vi "Loop_SM.vi"() -> ()   [LabVIEW 2017, in "Arm.lvlib"]
uses:
  Arm.lvlib
  CLUSTER_CMD_SM_Lift_Rotate.ctl
  ENUM_SM_Rotate_Positions.ctl
  _SHARE ALL/TypeDef Share All/CLUSTER_TalonInput.ctl
  System Drivers/Phoenix-LabVIEW/Motor Controller/Controls/CTRE_Phoenix_MotorControl_ControlMode.ctl
  TypeDef/CLUSTER_PID.ctl
  ENUM_SM_State.ctl
  CLUSTER_ACT_Lift Output.ctl
  _SHARE ALL/RoboRio Share All/SRX Share All/TypeDefs SRX/Cluster_SRX_General Data.ctl
  _SHARE ALL/RoboRio Share All/SRX Share All/TypeDefs SRX/Cluster_SRX_Common Runtime Data.ctl
  _SHARE ALL/RoboRio Share All/SRX Share All/TypeDefs SRX/Cluster_SRX_Error Calculations.ctl
  _SHARE ALL/RoboRio Share All/SRX Share All/TypeDefs SRX/Cluster_SRX_Voltage Out Data.ctl
  _SHARE ALL/RoboRio Share All/SRX Share All/TypeDefs SRX/Cluster_SRX_Sensor Out Data.ctl
  _SHARE ALL/RoboRio Share All/SRX Share All/TypeDefs SRX/Cluster_SRX_Sensor Quad Data.ctl
  _SHARE ALL/RoboRio Share All/SRX Share All/TypeDefs SRX/Cluster_SRX_Analog In Data.ctl
  _SHARE ALL/RoboRio Share All/SRX Share All/TypeDefs SRX/Cluster_SRX_PWM Sensor Data.ctl
  _SHARE ALL/RoboRio Share All/SRX Share All/TypeDefs SRX/Cluster_SRX_F and R Limit Indicators.ctl
  ENUM_SM_Action.ctl
  Globals/Global_Device_IDs.vi
  _SHARE ALL/Global Share All/Global_STOP.vi
  Global_CMD.vi
  Global_ACT Write_Data Out.vi
  Global_SM Write_Data Out.vi
panel:
  out "State":T1
  out "SM Output":T2 {"Talon Mode" items=["PercentOutput"=0, "Position"=1, "Velocity"=2, "Current"=3, "Follower"=5, "MotionProfile"=6, "MotionMagic"=7, "MotionMagicArc"=8, "MotionProfileArc"=10, "Disabled"=15]}
  out "SM CMD Input":T5={"Enable System"=TRUE, "Rotate Position"=enum."Neutral: 3340", "Manual Velocity"=0.0, "Manual Mode"=FALSE, "Manual Override"=FALSE}
  out "Cycle Time (S)":dbl format="%.3g"
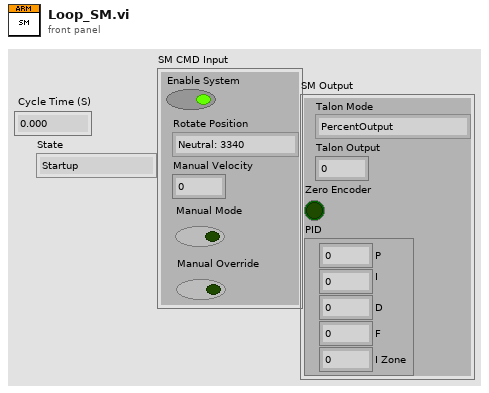
[diagram p1: front panel]
types:
  T1 = typedef "Arm.lvlib/ENUM_SM_State.ctl" = enum16{"Startup", "Idle", "F_Manual", "Manual", "Position - Moving", "Position - Holding", "Shutdown"}
  T2 = typedef "CLUSTER_TalonInput.ctl" = cluster{"Talon Mode":T3, "Talon Output":dbl, "Zero Encoder":bool, "PID":T4}
  T3 = typedef "CTRE_Phoenix_MotorControl_ControlMode.ctl" = u16
  T4 = typedef "CLUSTER_PID.ctl" = cluster{"P":dbl, "I":dbl, "D":dbl, "F":dbl, "I Zone":dbl}
  T5 = typedef "Arm.lvlib/CLUSTER_CMD_SM_Lift_Rotate.ctl" = cluster{"Enable System":bool, "Rotate Position":T6, "Manual Velocity":dbl, "Manual Mode":bool, "Manual Override":bool}
  T6 = typedef "Arm.lvlib/ENUM_SM_Rotate_Positions.ctl" = enum16{"Neutral: 3340", "Pickup: 0", "Switch: 0", "Scale: 0", "Climb: 0"}
  T7 = typedef "Arm.lvlib/CLUSTER_ACT_Lift Output.ctl" = cluster{"Device Info Out":T8, "Common Runtime Data Out":T9, "Quad Sensor Data Out":T13, "Analog Sensor Data Out":T14, "PWM Data Out":T15, "Hard Limits Out":T16}
  T8 = typedef "Cluster_SRX_General Data.ctl" = cluster{"Device ID":i32, "Firmware Version":i32, "Inverted?":bool, "Has Reset Occurred?":bool}
  T9 = typedef "Cluster_SRX_Common Runtime Data.ctl" = cluster{"Calc":T10, "Voltage ":T11, "Sensor":T12, "Current":dbl, "Temp":dbl}
  T10 = typedef "Cluster_SRX_Error Calculations.ctl" = cluster{"Error":i32, "D-Error":dbl, "I-Acc":dbl}
  T11 = typedef "Cluster_SRX_Voltage Out Data.ctl" = cluster{"Percent":dbl, "Output":dbl, "Bus":dbl}
  T12 = typedef "Cluster_SRX_Sensor Out Data.ctl" = cluster{"Pos":i32, "Vel":i32}
  T13 = typedef "Cluster_SRX_Sensor Quad Data.ctl" = cluster{"Position":i32, "Velocity":i32, "Quad A Pin":bool, "Quad B Pin":bool, "Quad Idx Pin":bool}
  T14 = typedef "Cluster_SRX_Analog In Data.ctl" = cluster{"WithOv":i32, "Raw":i32, "Velocity":i32}
  T15 = typedef "Cluster_SRX_PWM Sensor Data.ctl" = cluster{"Position":i32, "Velocity":i32, "High(us)":i32, "Period(us)":i32}
  T16 = typedef "Cluster_SRX_F and R Limit Indicators.ctl" = cluster{"Forward Closed?":bool, "Reverse Closed?":bool}
  T17 = typedef "Arm.lvlib/ENUM_SM_Action.ctl" = enum16{"No Action", "Reset Time", "Reset All", "Reset Encoder", "F_Manual", "Manual", "Position", "Set PID 1", "Disable Motor"}
  T18 = typedef "CLUSTER_Arm_Device_IDs.ctl" = cluster{"Master":T19, "Slave":T19, "Up PIDF":T27, "Down PIDF":T27}
  T19 = typedef "CLUSTER_Talon_Setup.ctl" = cluster{"Open Data":T20, "Current Config Data":T21, "Sensor Config":T22, "Hard Limits":T24, "Motion Magic Config Data":T26, "PIDF":T27, "Maximum Integral Accumulator Value":dbl, "AllowableClosedLoop":i32, "Limits":T28, "Output Config":T29}
  T20 = typedef "Cluster_SRX_OPEN Data.ctl" = cluster{"SRX ID":u8, "Invert Output":bool}
  T21 = typedef "Cluster_SRX_Current Config.ctl" = cluster{"Enable Current Limit?":bool, "Peak Current (Amps)":i32, "Peak Current Maximum Duration (ms)":i32, "Continuous Current Limit (Amps)":i32}
  T22 = typedef "Cluster_SRX_Sensor Config.ctl" = cluster{"Feedback Device":T23, "PhaseSensor":bool}
  T23 = typedef "CTRE_Phoenix_MotorControl_FeedbackDevice.ctl" = i8
  T24 = typedef "Cluster_SRX_Config Hard Limits.ctl" = cluster{"Fwd Enable":bool, "Rev Enable":bool, "Fwd NO-NC":T25, "Rev NO-NC":T25}
  T25 = typedef "CTRE_Phoenix_MotorControl_LimitSwitchNormal.ctl" = enum16{"Normally Open", "Normally Closed", "Disabled"}
  T26 = typedef "Cluster_SRX_Motion Magic Config Data.ctl" = cluster{"Cruise Velocity":i32, "Acceleration":i32}
  T27 = typedef "Cluster_SRX_PIDF.ctl" = cluster{"P":dbl, "I":dbl, "D":dbl, "F":dbl, "I Zone":dbl}
  T28 = typedef "Cluster_SRX_Config Soft Limits.ctl" = cluster{"Max":i32, "Min":i32, "Max Enable":bool, "Min Enable":bool}
  T29 = typedef "Cluster_SRX_Config Voltage Output.ctl" = cluster{"Invert?":bool, "Neutral Mode":T30, "Deadband (-1to1)":dbl, "Ramp Time Off to Full (S)":dbl, "Peak  (-1to1)":T31, "Nominal  (-1to1)":T31}
  T30 = typedef "CTRE_Phoenix_MotorControl_NeutralMode.ctl" = enum8{"EEPROMSetting", "Override to Coast", "Override to Brake"}
  T31 = typedef "Cluster_SRX_Forward and Reverse.ctl" = cluster{"Forward":dbl, "Reverse":dbl}
  T32 = cluster{"State":T1, "Previous State":T1, "Current Time":timestamp, "Previous Time":timestamp, "Start Time":timestamp, "Target Time (ms)":u32, "Cycle Time(S)":dbl, "Arm_Output":T7, "SM CMD Input":T5, "SM Output":T2, "Arm Setup":T18, "Manual Counter":i32}
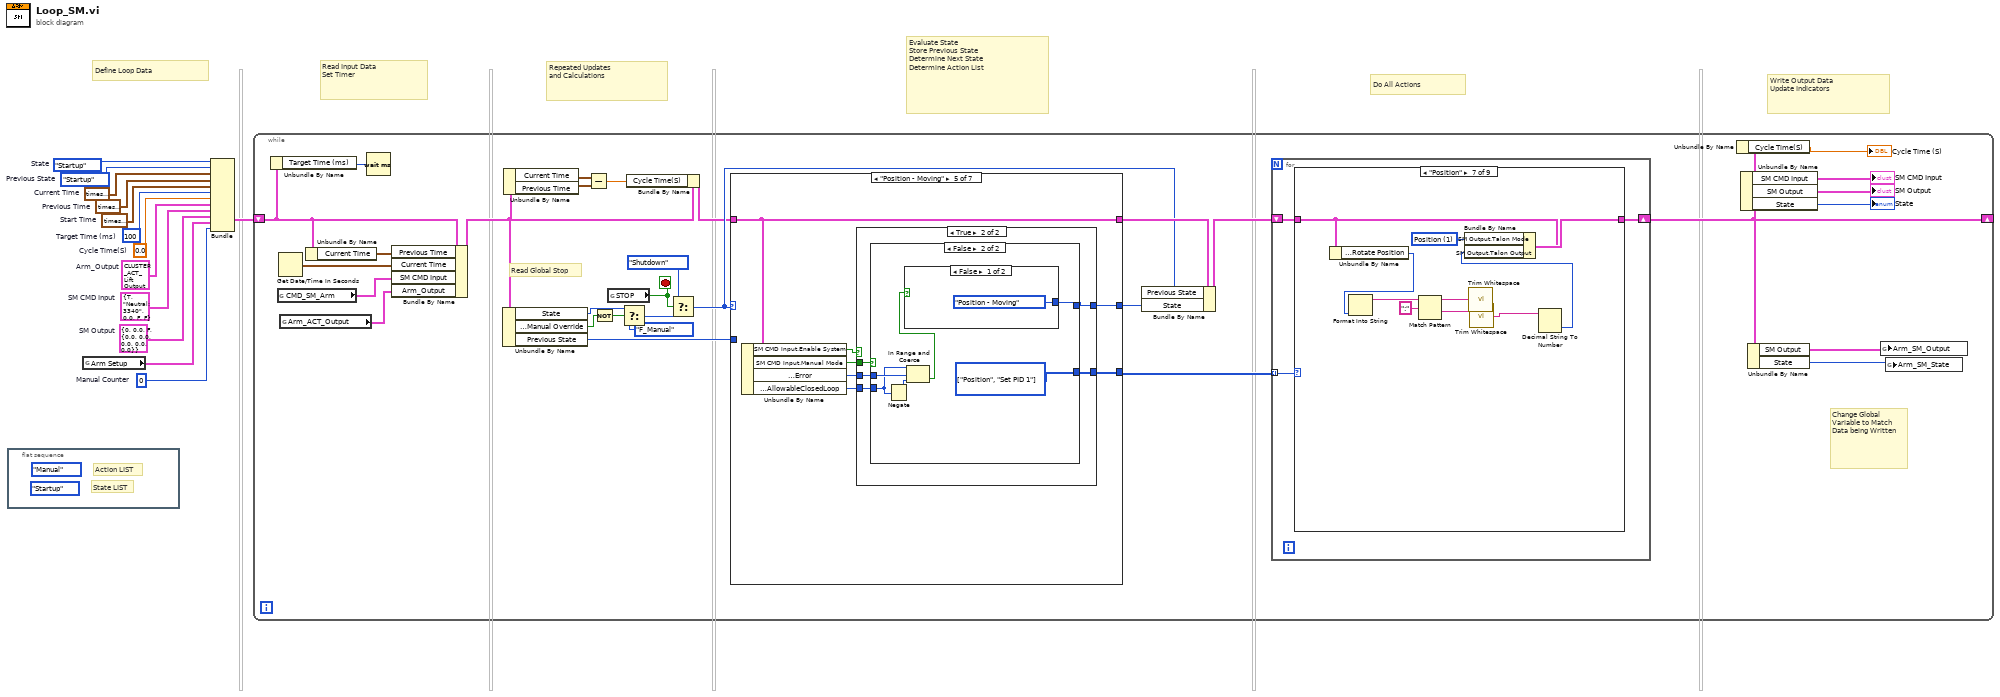
[diagram p0: block diagram]
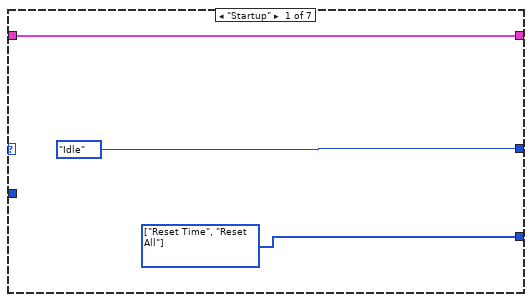
[diagram p2: hidden frame]
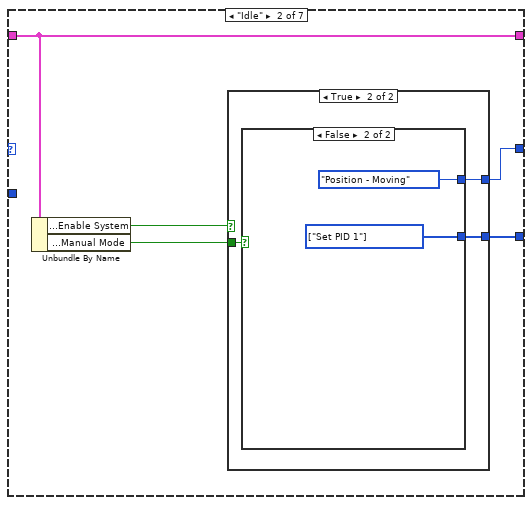
[diagram p3: hidden frame]
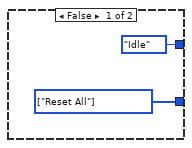
[diagram p4: hidden frame]
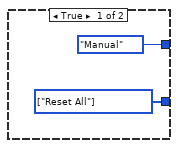
[diagram p5: hidden frame]
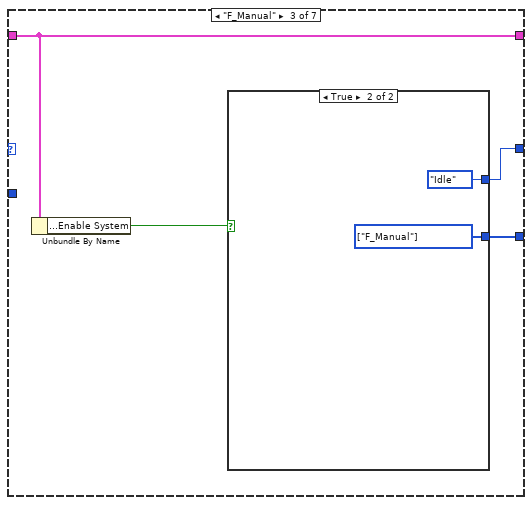
[diagram p6: hidden frame]
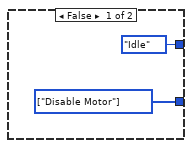
[diagram p7: hidden frame]
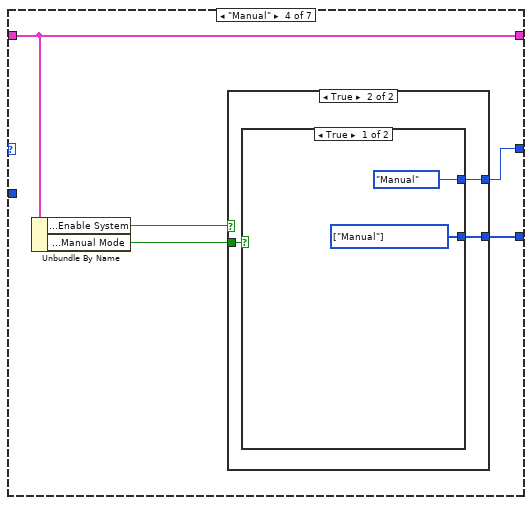
[diagram p8: hidden frame]
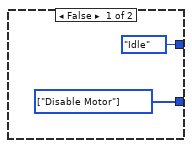
[diagram p9: hidden frame]
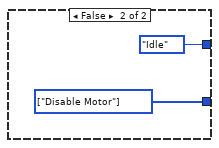
[diagram p10: hidden frame]
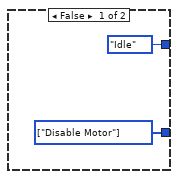
[diagram p11: hidden frame]
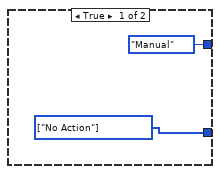
[diagram p12: hidden frame]
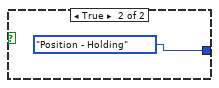
[diagram p13: hidden frame]
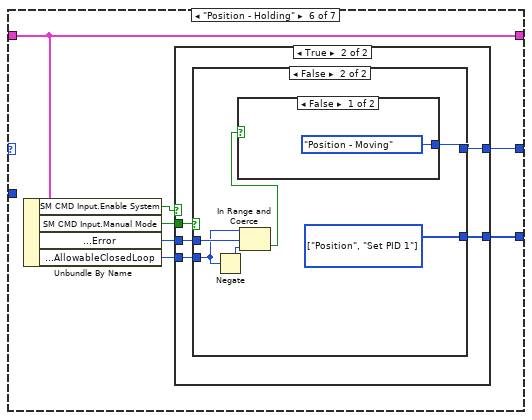
[diagram p14: hidden frame]
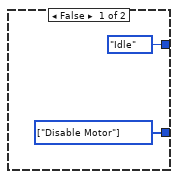
[diagram p15: hidden frame]
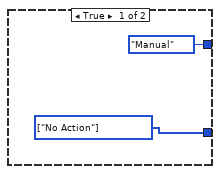
[diagram p16: hidden frame]
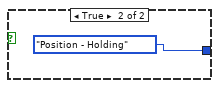
[diagram p17: hidden frame]
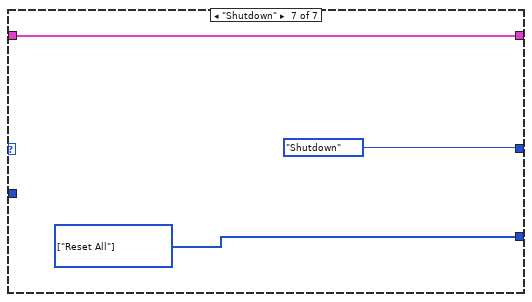
[diagram p18: hidden frame]
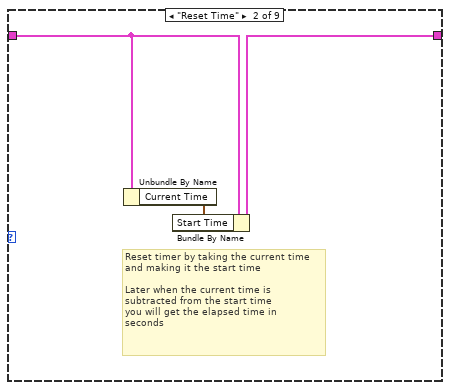
[diagram p20: hidden frame]
diagram:
  w1 = 0  # Manual Counter
  w3 = T2 {"Talon Mode"=0, "Talon Output"=0.0, "Zero Encoder"=FALSE, "PID"={"P"=0.0, "I"=0.0, "D"=0.0, "F"=0.0, "I Zone"=0.0}}  # SM Output
  w4 = T5 {"Enable System"=TRUE, "Rotate Position"=enum."Neutral: 3340", "Manual Velocity"=0.0, "Manual Mode"=FALSE, "Manual Override"=FALSE}  # SM CMD Input
  w5 = T7 {"Device Info Out"={"Device ID"=0, "Firmware Version"=0, "Inverted?"=FALSE, "Has Reset Occurred?"=FALSE}, "Common Runtime Data Out"={"Calc"={"Error"=0, "D-Error"=0.0, "I-Acc"=0.0}, "Voltage "={"Percent"=0.0, "Output"=0.0, "Bus"=0.0}, "Sensor"={"Pos"=0, "Vel"=0}, "Current"=0.0, "Temp"=0.0}, "Quad Sensor Data Out"={"Position"=0, "Velocity"=0, "Quad A Pin"=FALSE, "Quad B Pin"=FALSE, "Quad Idx Pin"=FALSE}, "Analog Sensor Data Out"={"WithOv"=0, "Raw"=0, "Velocity"=0}, "PWM Data Out"={"Position"=0, "Velocity"=0, "High(us)"=0, "Period(us)"=0}, "Hard Limits Out"={"Forward Closed?"=FALSE, "Reverse Closed?"=FALSE}}  # Arm_Output
  w6 = 0.0  # Cycle Time(S)
  w7 = ENUM_SM_State."Startup"  # Previous State
  w8 = timestamp(0 s since 1904-01-01)  # Previous Time
  w9 = u32 100  # Target Time (ms)
  w10 = timestamp(0 s since 1904-01-01)  # Start Time
  w11 = timestamp(0 s since 1904-01-01)  # Current Time
  w12 = ENUM_SM_State."Startup"  # State
  # "Define Loop Data"
  # "Repeated Updates\nand Calculations"
  # "Read Input Data\nSet Timer"
  # "Evaluate State\nStore Previous State\nDetermine Next State\nDetermine Action List"
  # "Do All Actions"
  # "Write Output Data\nUpdate Indicators"
  n1 = flat-sequence {
    frame #0 {
      (unwired) ENUM_SM_State."Startup" ("State")
      (unwired) ENUM_SM_Action."Manual" ("Action")
      # "State LIST"
      # "Action LIST"
    }
  }
  n2 = global read "Global_Device_IDs.vi" "Arm Setup"() -> (w2:T18)
  n3 = Bundle("State"=w12, "Previous State"=w7, "Current Time"=w11, "Previous Time"=w8, "Start Time"=w10, "Target Time (ms)"=w9, "Cycle Time(S)"=w6, "Arm_Output"=w5, "SM CMD Input"=w4, "SM Output"=w3, "Arm Setup"=w2, "Manual Counter"=w1) -> (w13:T32)  [unwired: 1 in]
  n4 = while {
    shift-right: [w35] -> _
    shift-left: w13 -> [w37]
    stop <- w41 stop-if-true
    # "Change Global\nVariable to Match\nData being Written"
    # "Read Global Stop"
    n5 = Unbundle By Name(w37) -> ("Target Time (ms)"=w39:u32)
    n6 = global read "Global_CMD.vi" "CMD_SM_Arm"() -> (w27:T5)
    n7 = Get Date/Time In Seconds() -> (seconds since 1Jan1904=w44:timestamp)
    n8 = global read "Global_ACT Write_Data Out.vi" "Arm_ACT_Output"() -> (w26:T7)
    n9 = Unbundle By Name(w37) -> ("Current Time"=w38:timestamp)
    n10 = Wait (ms)(milliseconds to wait=w39) -> ()  [unwired: 1 out]
    n11 = Bundle By Name(cluster=w37, "Previous Time"=w38, "Current Time"=w44, "SM CMD Input"=w27, "Arm_Output"=w26) -> (w31:T32)
    n12 = Unbundle By Name(w31) -> ("State"=w17:T1, "SM CMD Input.Manual Override"=w18:bool, "Previous State"=w19:T1)
    n13 = Unbundle By Name(w31) -> ("Current Time"=w32:timestamp, "Previous Time"=w33:timestamp)
    n14 = Subtract(x=w32, y=w33) -> (x-y=w29:dbl)
    n15 = Not(x=w18) -> (.not. x?=w14:bool)
    n16 = global read "Global_STOP.vi" "STOP"() -> (w41:bool)
    n17 = Select(t=w17, s=w14, f=ENUM_SM_State."F_Manual") -> (s? t:f=w15:T1)
    n18 = Bundle By Name(cluster=w31, "Cycle Time(S)"=w29) -> (w30:T32)
    n19 = Select(t=ENUM_SM_State."Shutdown" ("State"), s=w41, f=w15) -> (s? t:f=w36:T1)
    n20 = case shown="\"Position - Moving\"" w36 {
      tunnel: w30 -> [w47 w52 w65 w74 w90 w114 w134]
      tunnel: [w47 w52 w65 w74 w90 w114 w134] -> w42
      tunnel: [w46 w48 w62 w70 w86 w110 w133] -> w28
      tunnel: [ENUM_SM_State."Idle" ("State") w49 w63 w71 w85 w109 ENUM_SM_State."Shutdown" ("State")] -> w25
      tunnel: w19 -> [_ _ _ _ _ _ _]
      frame "Startup" {
        w46 = T17[] [enum."Reset Time", enum."Reset All"] items=["No Action", "Reset Time", "Reset All", "Reset Encoder", "F_Manual", "Manual", "Position", "Set PID 1", "Disable Motor"] ("Actions")
      }
      frame "Idle" {
        n21 = Unbundle By Name(w52) -> ("SM CMD Input.Enable System"=w51:bool, "SM CMD Input.Manual Mode"=w50:bool)
        n22 = case shown="True" w51 {
          tunnel: w50 -> [_ w57]
          tunnel: [ENUM_SM_State."Idle" ("State") w56] -> w49
          tunnel: [w53 w55] -> w48
          frame False {
            w53 = T17[] [enum."Reset All"] items=["No Action", "Reset Time", "Reset All", "Reset Encoder", "F_Manual", "Manual", "Position", "Set PID 1", "Disable Motor"] ("Actions")
          }
          frame True {
            n23 = case shown="False" w57 {
              tunnel: [ENUM_SM_State."Manual" ("State") ENUM_SM_State."Position - Moving" ("State")] -> w56
              tunnel: [w58 w60] -> w55
              frame True {
                w58 = T17[] [enum."Reset All"] items=["No Action", "Reset Time", "Reset All", "Reset Encoder", "F_Manual", "Manual", "Position", "Set PID 1", "Disable Motor"] ("Actions")
              }
              frame False {
                w60 = T17[] [enum."Set PID 1"] items=["No Action", "Reset Time", "Reset All", "Reset Encoder", "F_Manual", "Manual", "Position", "Set PID 1", "Disable Motor"] ("Actions")
              }
            }
          }
        }
      }
      frame "F_Manual" {
        n24 = Unbundle By Name(w65) -> ("SM CMD Input.Enable System"=w64:bool)
        n25 = case shown="True" w64 {
          tunnel: [ENUM_SM_State."Idle" ("State") ENUM_SM_State."Idle" ("State")] -> w63
          tunnel: [w66 w68] -> w62
          frame False {
            w66 = T17[] [enum."Disable Motor"] items=["No Action", "Reset Time", "Reset All", "Reset Encoder", "F_Manual", "Manual", "Position", "Set PID 1", "Disable Motor"] ("Actions")
          }
          frame True {
            w68 = T17[] [enum."F_Manual"] items=["No Action", "Reset Time", "Reset All", "Reset Encoder", "F_Manual", "Manual", "Position", "Set PID 1", "Disable Motor"] ("Actions")
          }
        }
      }
      frame "Manual" {
        n26 = Unbundle By Name(w74) -> ("SM CMD Input.Enable System"=w73:bool, "SM CMD Input.Manual Mode"=w72:bool)
        n27 = case shown="True" w73 {
          tunnel: w72 -> [_ w79]
          tunnel: [ENUM_SM_State."Idle" ("State") w78] -> w71
          tunnel: [w75 w77] -> w70
          frame False {
            w75 = T17[] [enum."Disable Motor"] items=["No Action", "Reset Time", "Reset All", "Reset Encoder", "F_Manual", "Manual", "Position", "Set PID 1", "Disable Motor"] ("Actions")
          }
          frame True {
            n28 = case shown="True" w79 {
              tunnel: [ENUM_SM_State."Manual" ("State") ENUM_SM_State."Idle" ("State")] -> w78
              tunnel: [w80 w82] -> w77
              frame True {
                w80 = T17[] [enum."Manual"] items=["No Action", "Reset Time", "Reset All", "Reset Encoder", "F_Manual", "Manual", "Position", "Set PID 1", "Disable Motor"] ("Actions")
              }
              frame False {
                w82 = T17[] [enum."Disable Motor"] items=["No Action", "Reset Time", "Reset All", "Reset Encoder", "F_Manual", "Manual", "Position", "Set PID 1", "Disable Motor"] ("Actions")
              }
            }
          }
        }
      }
      frame "Position - Moving" {
        n29 = Unbundle By Name(w90) -> ("SM CMD Input.Enable System"=w84:bool, "SM CMD Input.Manual Mode"=w89:bool, "Arm_Output.Common Runtime Data Out.Calc.Error"=w88:i32, "Arm Setup.Master.AllowableClosedLoop"=w87:i32)
        n30 = case shown="True" w84 {
          tunnel: w89 -> [_ w97]
          tunnel: w88 -> [_ w96]
          tunnel: w87 -> [_ w95]
          tunnel: [w91 w94] -> w86
          tunnel: [ENUM_SM_State."Idle" ("State") w93] -> w85
          frame False {
            w91 = T17[] [enum."Disable Motor"] items=["No Action", "Reset Time", "Reset All", "Reset Encoder", "F_Manual", "Manual", "Position", "Set PID 1", "Disable Motor"] ("Actions")
          }
          frame True {
            n31 = case shown="False" w97 {
              tunnel: w96 -> [_ w105]
              tunnel: w95 -> [_ w104]
              tunnel: [w98 w101] -> w94
              tunnel: [ENUM_SM_State."Manual" ("State") w100] -> w93
              frame True {
                w98 = T17[] [enum."No Action"] items=["No Action", "Reset Time", "Reset All", "Reset Encoder", "F_Manual", "Manual", "Position", "Set PID 1", "Disable Motor"] ("Actions")
              }
              frame False {
                w101 = T17[] [enum."Position", enum."Set PID 1"] items=["No Action", "Reset Time", "Reset All", "Reset Encoder", "F_Manual", "Manual", "Position", "Set PID 1", "Disable Motor"] ("Actions")
                n32 = Negate(x=w104) -> (-x=w103:i32)
                n33 = In Range and Coerce(upper limit=w104, x=w105, lower limit=w103) -> (In Range?=w102:bool)  [unwired: 1 out]
                n34 = case shown="False" w102 {
                  tunnel: [ENUM_SM_State."Position - Moving" ("State") ENUM_SM_State."Position - Holding" ("State")] -> w100
                  frame False {
                  }
                  frame True {
                  }
                }
              }
            }
          }
        }
      }
      frame "Position - Holding" {
        n35 = Unbundle By Name(w114) -> ("SM CMD Input.Enable System"=w108:bool, "SM CMD Input.Manual Mode"=w113:bool, "Arm_Output.Common Runtime Data Out.Calc.Error"=w112:i32, "Arm Setup.Master.AllowableClosedLoop"=w111:i32)
        n36 = case shown="True" w108 {
          tunnel: w113 -> [_ w121]
          tunnel: w112 -> [_ w120]
          tunnel: w111 -> [_ w119]
          tunnel: [w115 w118] -> w110
          tunnel: [ENUM_SM_State."Idle" ("State") w117] -> w109
          frame False {
            w115 = T17[] [enum."Disable Motor"] items=["No Action", "Reset Time", "Reset All", "Reset Encoder", "F_Manual", "Manual", "Position", "Set PID 1", "Disable Motor"] ("Actions")
          }
          frame True {
            n37 = case shown="False" w121 {
              tunnel: w120 -> [_ w129]
              tunnel: w119 -> [_ w128]
              tunnel: [w122 w125] -> w118
              tunnel: [ENUM_SM_State."Manual" ("State") w124] -> w117
              frame True {
                w122 = T17[] [enum."No Action"] items=["No Action", "Reset Time", "Reset All", "Reset Encoder", "F_Manual", "Manual", "Position", "Set PID 1", "Disable Motor"] ("Actions")
              }
              frame False {
                w125 = T17[] [enum."Position", enum."Set PID 1"] items=["No Action", "Reset Time", "Reset All", "Reset Encoder", "F_Manual", "Manual", "Position", "Set PID 1", "Disable Motor"] ("Actions")
                n38 = Negate(x=w128) -> (-x=w127:i32)
                n39 = In Range and Coerce(upper limit=w128, x=w129, lower limit=w127) -> (In Range?=w126:bool)  [unwired: 1 out]
                n40 = case shown="False" w126 {
                  tunnel: [ENUM_SM_State."Position - Moving" ("State") ENUM_SM_State."Position - Holding" ("State")] -> w124
                  frame False {
                  }
                  frame True {
                  }
                }
              }
            }
          }
        }
      }
      frame "Shutdown" {
        w133 = T17[] [enum."Reset All"] items=["No Action", "Reset Time", "Reset All", "Reset Encoder", "F_Manual", "Manual", "Position", "Set PID 1", "Disable Motor"] ("Actions")
      }
    }
    n41 = Bundle By Name(cluster=w42, "Previous State"=w36, "State"=w25) -> (w43:T32)
    n42 = for {
      tunnel: w28 -> [w137] mode=indexing
      shift-right: [w136] -> w35
      shift-left: w43 -> [w135]
      n43 = case shown="\"Position\"" w137 {
        tunnel: w135 -> [w138 w141 w147 w150 w151 w166 w197 w200 w204]
        tunnel: [w138 w140 w146 w149 w157 w173 w198 w201 w203] -> w136
        frame "No Action" {
        }
        frame "Reset Time" {
          # "Reset timer by taking the current time\nand making it the start time\n\nLater when the current time is \nsubtracted from the start time\nyou will get the elapsed time in \nseconds"
          n44 = Unbundle By Name(w141) -> ("Current Time"=w139:timestamp)
          n45 = Bundle By Name(cluster=w141, "Start Time"=w139) -> (w140:T32)
        }
        frame "Reset All" {
          w145 = T3 15 items=["PercentOutput"=0, "Position"=1, "Velocity"=2, "Current"=3, "Follower"=5, "MotionProfile"=6, "MotionMagic"=7, "MotionMagicArc"=8, "MotionProfileArc"=10, "Disabled"=15] ("SM Output.Talon Mode")
          n46 = Bundle By Name(cluster=w147, "SM Output.Talon Mode"=w145, "SM Output.Talon Output"=0.0, "SM Output.Zero Encoder"=FALSE, "Manual Counter"=0) -> (w146:T32)
        }
        frame "Reset Encoder" {
          n47 = Bundle By Name(cluster=w150, "SM Output.Zero Encoder"=TRUE) -> (w149:T32)
        }
        frame "F_Manual" {
          n48 = Unbundle By Name(w151) -> ("SM CMD Input.Manual Velocity"=w156:dbl, "Arm Setup.Master.Output Config.Deadband (-1to1)"=w160:dbl, "Arm_Output.Common Runtime Data Out.Sensor.Pos"=w152:i32)
          n49 = Negate(x=w160) -> (-x=w159:dbl)
          n50 = In Range and Coerce(upper limit=w160, x=w156, lower limit=w159) -> (In Range?=w158:bool)  [unwired: 1 out]
          n51 = case shown="True" w158 {
            tunnel: w156 -> [_ w164]
            tunnel: [w162 w165] -> w155
            tunnel: [w161 w164] -> w154
            tunnel: [w161 0] -> w153
            tunnel: w152 -> [_ _]
            frame True {
              w161 = 0
              w162 = T3 15 items=["PercentOutput"=0, "Position"=1, "Velocity"=2, "Current"=3, "Follower"=5, "MotionProfile"=6, "MotionMagic"=7, "MotionMagicArc"=8, "MotionProfileArc"=10, "Disabled"=15] ("SM Output.Talon Mode")
            }
            frame False {
              w165 = T3 0 items=["PercentOutput"=0, "Position"=1, "Velocity"=2, "Current"=3, "Follower"=5, "MotionProfile"=6, "MotionMagic"=7, "MotionMagicArc"=8, "MotionProfileArc"=10, "Disabled"=15] ("SM Output.Talon Mode")
            }
          }
          n52 = Bundle By Name(cluster=w151, "SM Output.Talon Mode"=w155, "SM Output.Talon Output"=w154, "Manual Counter"=w153) -> (w157:T32)
        }
        frame "Manual" {
          n53 = Unbundle By Name(w166) -> ("SM CMD Input.Manual Velocity"=w172:dbl, "Arm Setup.Master.Output Config.Deadband (-1to1)"=w176:dbl, "Arm_Output.Common Runtime Data Out.Sensor.Pos"=w168:i32, "Manual Counter"=w167:i32)
          n54 = Negate(x=w176) -> (-x=w175:dbl)
          n55 = In Range and Coerce(upper limit=w176, x=w172, lower limit=w175) -> (In Range?=w174:bool)  [unwired: 1 out]
          n56 = case shown="True" w174 {
            tunnel: w172 -> [_ w187]
            tunnel: [w185 w188] -> w171
            tunnel: [w177 w187] -> w170
            tunnel: [1 0] -> w169
            tunnel: w168 -> [w184 _]
            tunnel: w167 -> [w183 _]
            tunnel: w166 -> [w180 _]
            frame True {
              w185 = T3 1 items=["PercentOutput"=0, "Position"=1, "Velocity"=2, "Current"=3, "Follower"=5, "MotionProfile"=6, "MotionMagic"=7, "MotionMagicArc"=8, "MotionProfileArc"=10, "Disabled"=15] ("SM Output.Talon Mode")
              n57 = Unbundle By Name(w180) -> ("SM Output.Talon Output"=w179:dbl)
              n58 = Greater Than 0?(x=w183) -> (x > 0?=w182:bool)
              n59 = Not(x=w182) -> (.not. x?=w181:bool)
              n60 = Select(t=w184, s=w181, f=w179) -> (s? t:f=w177:dbl)
            }
            frame False {
              w188 = T3 0 items=["PercentOutput"=0, "Position"=1, "Velocity"=2, "Current"=3, "Follower"=5, "MotionProfile"=6, "MotionMagic"=7, "MotionMagicArc"=8, "MotionProfileArc"=10, "Disabled"=15] ("SM Output.Talon Mode")
            }
          }
          n61 = Bundle By Name(cluster=w166, "SM Output.Talon Mode"=w171, "SM Output.Talon Output"=w170, "Manual Counter"=w169) -> (w173:T32)
        }
        frame "Position" {
          w189 = T3 1 items=["PercentOutput"=0, "Position"=1, "Velocity"=2, "Current"=3, "Follower"=5, "MotionProfile"=6, "MotionMagic"=7, "MotionMagicArc"=8, "MotionProfileArc"=10, "Disabled"=15] ("SM Output.Talon Mode")
          n62 = Unbundle By Name(w197) -> ("SM CMD Input.Rotate Position"=w191:T6)
          n63 = Format Into String(w191) -> (resulting string=w196:string)  [unwired: 3 in, 1 out]
          n64 = Match Pattern(string=w196, regular expression=":") -> (before substring=w194:string, after substring=w193:string)  [unwired: 1 in, 2 out]
          n65 = call <vilib>:"Trim Whitespace.vi"("string"=w194) -> ()  [unwired: 1 in, 1 out]
          n66 = call <vilib>:"Trim Whitespace.vi"("string"=w193) -> ("trimmed string"=w192:string)  [unwired: 1 in]
          n67 = Decimal String To Number(string=w192) -> (number=w190:i32)  [unwired: 2 in, 1 out]
          n68 = Bundle By Name(cluster=w197, "SM Output.Talon Mode"=w189, "SM Output.Talon Output"=w190) -> (w198:T32)
        }
        frame "Set PID 1" {
          n69 = Unbundle By Name(w200) -> ("Arm Setup.Master.PIDF"=w199:T27)
          n70 = Bundle By Name(cluster=w200, "SM Output.PID"=w199) -> (w201:T32)
        }
        frame "Disable Motor" {
          w202 = T3 15 items=["PercentOutput"=0, "Position"=1, "Velocity"=2, "Current"=3, "Follower"=5, "MotionProfile"=6, "MotionMagic"=7, "MotionMagicArc"=8, "MotionProfileArc"=10, "Disabled"=15] ("SM Output.Talon Mode")
          n71 = Bundle By Name(cluster=w204, "SM Output.Talon Mode"=w202) -> (w203:T32)
        }
      }
    }
    n72 = Unbundle By Name(w35) -> ("Cycle Time(S)"=→"Cycle Time (S)":dbl)
    n73 = Unbundle By Name(w35) -> ("SM CMD Input"=→"SM CMD Input":T5, "SM Output"=→"SM Output":T2, "State"=→"State":T1)
    n74 = Unbundle By Name(w35) -> ("SM Output"=w23:T2, "State"=w24:T1)
    n75 = global write "Global_SM Write_Data Out.vi" "Arm_SM_Output"(w23) -> ()
    n76 = global write "Global_SM Write_Data Out.vi" "Arm_SM_State"(w24) -> ()
  }
